vi "AutoSetShooter.vi"(11 "Array":dbl[](array[numeric]) format="%0.3f") -> ()   [LabVIEW 2013]
uses:
  Shooter/Shooter Manual Control.ctl
  Shooter/Shooter Command.ctl
  Robot Global Data.vi
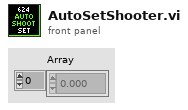
[diagram p1: front panel]
types:
  T1 = typedef "Shooter Manual Control.ctl" = cluster{"Command":T2, "Offset":dbl, "Trigger":bool, "Add":bool, "Release":bool, "Reset":bool, "Target Pressure":dbl, "Punch":bool, "AutoPunch":bool}
  T2 = typedef "Shooter Command.ctl" = enum16{"None", "Warmup", "Shoot", "Line Shoot", "Soft Shoot", "Toss"}
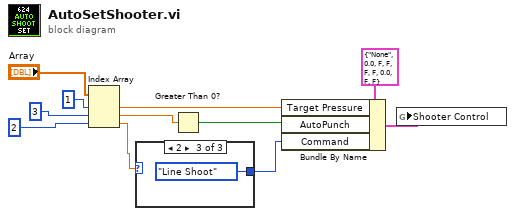
[diagram p0: block diagram]
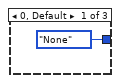
[diagram p2: hidden frame]
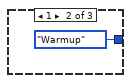
[diagram p3: hidden frame]
diagram:
  n1 = Index Array(array="Array", index #1=1 ("index"), index #2=3 ("index"), index #3=2 ("index")) -> (element #1=w7:dbl, element #2=w2:dbl, element #3=w5:dbl)
  n2 = case shown="2" w5 {
    tunnel: [Shooter_Command."None" ("Enum") Shooter_Command."Warmup" ("Enum") Shooter_Command."Line Shoot" ("Enum")] -> w6
    frame 0, Default {
    }
    frame 1 {
    }
    frame 2 {
    }
  }
  n3 = Greater Than 0?(x=w2) -> (x > 0?=w1:bool)
  n4 = Bundle By Name(cluster=T1 {"Command"=enum."None", "Offset"=0.0, "Trigger"=FALSE, "Add"=FALSE, "Release"=FALSE, "Reset"=FALSE, "Target Pressure"=0.0, "Punch"=FALSE, "AutoPunch"=FALSE} ("Shooter Manual Control"), "Target Pressure"=w7, "AutoPunch"=w1, "Command"=w6) -> (w8:T1)
  n5 = global write "Robot Global Data.vi" "Shooter Control"(w8) -> ()
